vi "Process.vi"(8 "error in (no error)":errorcluster, 10 "pound in":refnum<class "Pound.lvclass">, 11 "Qbus in":refnum<class "Qbus.lvclass">) -> (0 "error out":errorcluster)   [LabVIEW 2017, in "DataAccumulator.lvlib"]
doc: "This process combines waveforms from successive acquisitions to achieve the data block sizes configured in Systems Manager. The combined waveforms make up the data sets on which the Analysis process calculates features and spectral bands. Later, the Trigger and Alarm processes evaluate those feature values for operating state and alarm transitions."
uses:
  <vilib>/addons/InsightCM/Devices/Shared/Common/DataAccumulator/DataAccumulator.lvlib
  <vilib>/addons/Qbus/Qbus.lvclass
  <vilib>/NI/Software Watchdog/Pound/Pound.lvclass
  <vilib>/addons/TimerProcess/controls/taskType.ctl
  <vilib>/addons/InsightCM/Devices/Shared/Common/DataFlow/controls/Type.ctl
  <vilib>/addons/InsightCM/Devices/Shared/Common/DataAccumulator/controls/DataStoreOps.ctl
  <vilib>/addons/TraceLogger/TraceLogger.lvlib
  <vilib>/NI/Software Watchdog/Watchdog/Watchdog.lvclass
  <vilib>/addons/InsightCM/Devices/Shared/Common/DVRBuffer/DVRBuffer.lvlib
  <vilib>/addons/InsightCM/Devices/Shared/Common/DataFlow/DataFlow.lvlib
  <vilib>/addons/InsightCM/Utilities/GlobalConfiguration/GlobalConfiguration.lvlib
  <vilib>/addons/TimerProcess/TimerProcess.lvlib
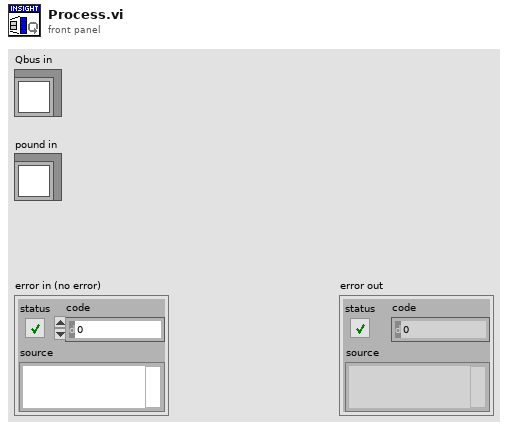
[diagram p1: front panel]
types:
  T1 = typedef "TimerProcess.lvlib/taskType.ctl" = enum16{"single", "repeat"}
  T2 = typedef "DataFlow.lvlib/Type.ctl" = enum16{"High Rate", "Low Rate", "Burst Mode"}
  T3 = typedef "DataAccumulator.lvlib/DataStoreOps.ctl" = enum16{"Reset", "Init", "Clear", "SetWfms", "GetWfms"}
  T4 = typedef "DataFlow.lvlib/Data.ctl" = cluster{"DataGroup":string, "Waveforms":T5, "Map":T6, "Type":T2}
  T5 = typedef "wfmSGL_DVR.ctl" = refnum<data-value>
  T6 = typedef "PointValueMap.lvlib/PointMap.ctl" = refnum<data-value>
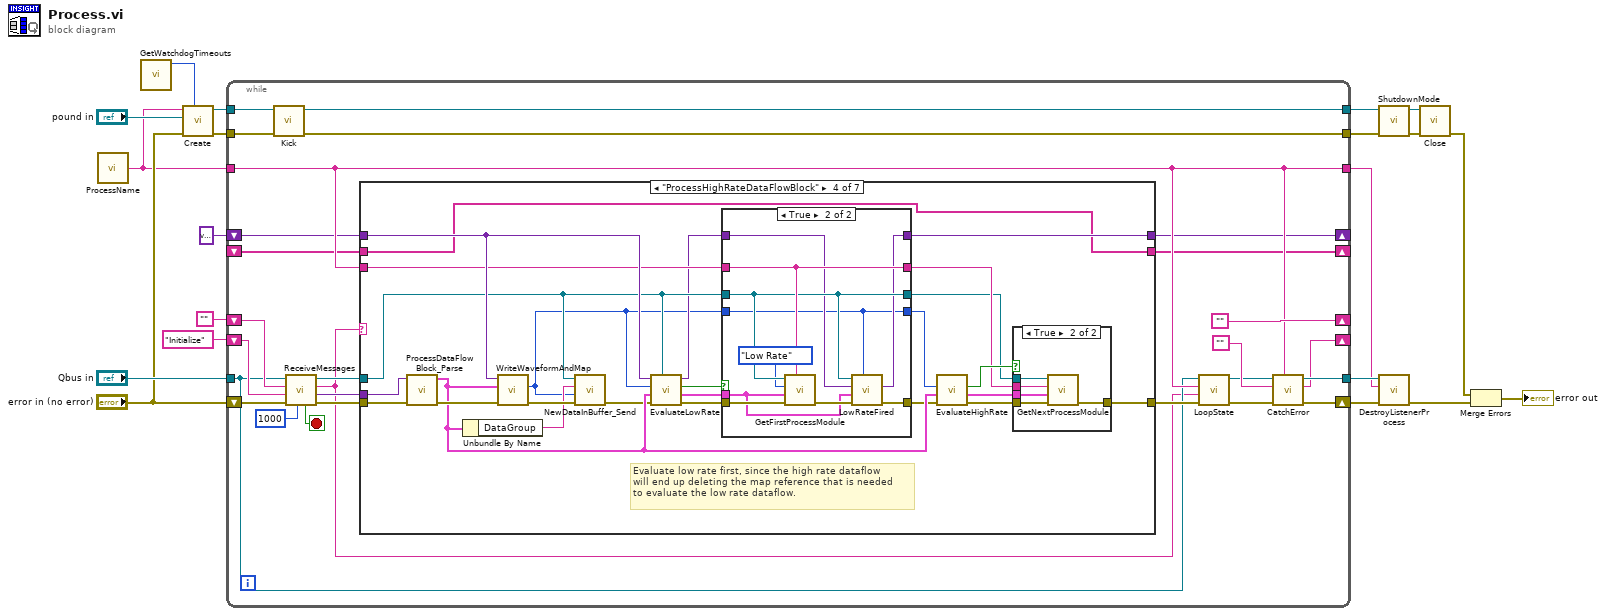
[diagram p0: block diagram]
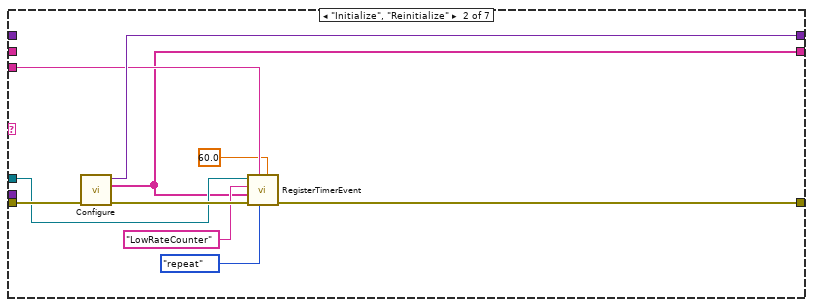
[diagram p3: hidden frame]
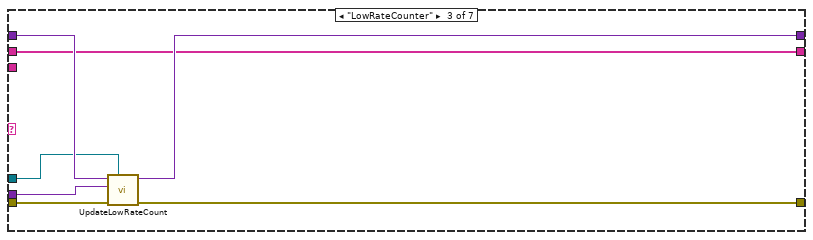
[diagram p4: hidden frame]
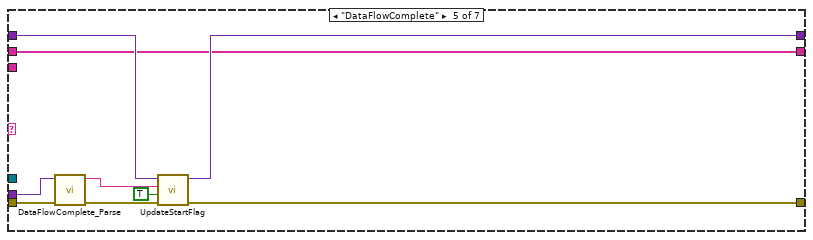
[diagram p7: hidden frame]
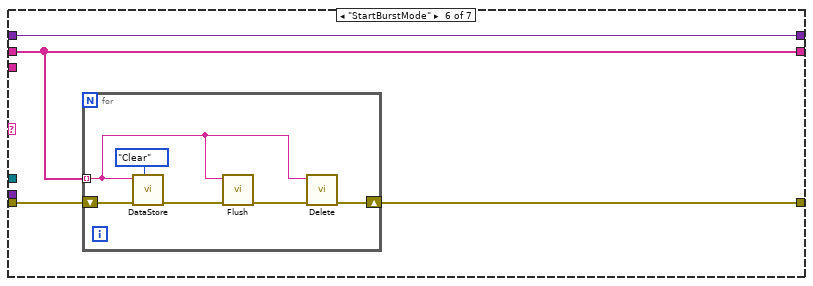
[diagram p8: hidden frame]
diagram:
  n1 = call <vilib>:"ProcessName.vi"() -> ("process name"=w1:string)  [unwired: 5 in]
  n2 = call <vilib>:"GetWatchdogTimeouts.vi"() -> ("software timeout"=w2:u32)  [unwired: 10 in, 1 out]
  n3 = call <vilib>:"Create.vi"("Execution Timeout (ms)"=w2, "error in (no error)"="error in (no error)", "Pound"="pound in", "Name"=w1) -> ("error out"=w10:errorcluster, "Watchdog"=w15:refnum<data-value>)  [unwired: 6 in]
  n4 = while {
    shift-right: [""] -> _
    shift-left: "" -> [w46]
    tunnel: "Qbus in" -> [w34]
    tunnel: w1 -> [w35]
    tunnel: [w39] -> w18
    tunnel: [w35] -> w17
    shift-right: [w37] -> _
    shift-left: "Initialize" -> [w41]
    tunnel: w15 -> [w33]
    tunnel: [w32] -> w12
    tunnel: w10 -> [w31]
    tunnel: [w29] -> w9
    shift-right: [w26] -> _
    shift-left: variant -> [w25]
    shift-right: [w40] -> w19
    shift-left: "error in (no error)" -> [w30]
    shift-right: [w22] -> _
    shift-left: _ -> [w21]
    stop <- w47 stop-if-true
    n5 = call <vilib>:"Kick.vi"("error in (no error)"=w31, "Watchdog"=w33) -> ("error out"=w29:errorcluster, "Watchdog"=w32:refnum<data-value>)  [unwired: 8 in]
    n6 = call <vilib>:"ReceiveMessages.vi"("timeout (1000)"=1000 ("milliseconds to wait"), "error in (no error)"=w30, "priority action"=w41, "default action"=w46, "Qbus in"=w34) -> ("error out"=w45:errorcluster, "message value"=w42:variant, "action"=w28:string, "Qbus out"=w43:refnum<class "Qbus.lvclass">, "exit"=w47:bool)  [unwired: 2 in]
    n7 = case shown="\"ProcessHighRateDataFlowBlock\"" w28 {
      tunnel: w45 -> [w50 w60 w63 w91 w118 w125 w135]
      tunnel: w43 -> [_ w56 w62 w75 _ _ _]
      tunnel: [w50 w57 w65 w76 w121 w124 w135] -> w36
      tunnel: w42 -> [_ _ w64 w90 w116 _ _]
      tunnel: w35 -> [_ w55 _ w81 _ _ _]
      tunnel: [w49 w59 w66 w74 w120 w126 w134] -> w26
      tunnel: w25 -> [w49 _ w67 w87 w122 w126 w134]
      tunnel: [w48 w51 w61 w68 w114 w123 w133] -> w22
      tunnel: w21 -> [w48 _ w61 w68 w114 w123 w133]
      frame "", Default {
      }
      frame "Initialize", "Reinitialize" {
        n8 = call <vilib>:"Configure.vi"("error in (no error)"=w60) -> ("error out"=w58:errorcluster, "groups"=w51:string[], "config"=w59:variant)  [unwired: 8 in]
        n9 = call <vilib>:"RegisterTimerEvent.vi"("interval (sec)"=60.0, "type"=taskType."repeat", "process name"=w55, "error in (no error)"=w58, "callback value"=w51, "callback action"="LowRateCounter", "qbus in"=w56) -> ("error out"=w57:errorcluster)  [unwired: 3 in, 1 out]
      }
      frame "LowRateCounter" {
        n10 = call <vilib>:"UpdateLowRateCount.vi"("Qbus in"=w62, "error in (no error)"=w63, "message value"=w64, "config"=w67) -> ("error out"=w65:errorcluster, "config out"=w66:variant)  [unwired: 6 in]
      }
      frame "ProcessHighRateDataFlowBlock" {
        # "Evaluate low rate first, since the high rate dataflow\nwill end up deleting the map reference that is needed\nto evaluate the low rate dataflow."
        n11 = call <vilib>:"ProcessDataFlowBlock_Parse.vi"("error in (no error)"=w91, "body"=w90) -> ("error out"=w88:errorcluster, "data"=w80:T4)  [unwired: 8 in]
        n12 = Unbundle By Name(w80) -> ("DataGroup"=w89:string)
        n13 = call <vilib>:"WriteWaveformAndMap.vi"("error in (no error)"=w88, "data"=w80, "config"=w87) -> ("error out"=w92:errorcluster, "block number"=w70:u32)  [unwired: 6 in, 1 out]
        n14 = call <vilib>:"NewDataInBuffer_Send.vi"("error in (no error)"=w92, "buffer location"=w70, "data group"=w89, "Qbus in"=w75) -> ("error out"=w79:errorcluster)  [unwired: 6 in, 1 out]
        n15 = call <vilib>:"EvaluateLowRate.vi"("Qbus"=w75, "error in (no error)"=w79, "data"=w80, "new block number"=w70, "config"=w87) -> ("error out"=w84:errorcluster, "new data"=w85:T4, "fire low rate data flow"=w86:bool, "config out"=w73:variant)  [unwired: 3 in]
        n16 = case shown="True" w86 {
          tunnel: w85 -> [_ w110]
          tunnel: w84 -> [w103 w113]
          tunnel: [w103 w111] -> w78
          tunnel: w75 -> [w100 w108]
          tunnel: w81 -> [w101 w109]
          tunnel: [w102 w106] -> w74
          tunnel: w73 -> [w102 w107]
          tunnel: [w101 w109] -> w72
          tunnel: [w100 w108] -> w71
          tunnel: w70 -> [w99 w105]
          tunnel: [w99 w105] -> w69
          frame False {
          }
          frame True {
            n17 = call <vilib>:"GetFirstProcessModule.vi"("originator"=w109, "error in (no error)"=w113, "data"=w110, "type"=Type."Low Rate", "Qbus in"=w108) -> ("error out"=w112:errorcluster)  [unwired: 5 in, 1 out]
            n18 = call <vilib>:"LowRateFired.vi"("new block number"=w105, "error in (no error)"=w112, "new data"=w110, "config in"=w107, "Qbus"=w108) -> ("error out"=w111:errorcluster, "config out"=w106:variant)  [unwired: 5 in]
          }
        }
        n19 = call <vilib>:"EvaluateHighRate.vi"("error in (no error)"=w78, "data in"=w80, "block number"=w69) -> ("error out"=w77:errorcluster, "data out"=w83:T4, "complete"=w82:bool)  [unwired: 6 in]
        n20 = case shown="True" w82 {
          tunnel: w72 -> [_ w98]
          tunnel: [w93 w95] -> w76
          tunnel: w71 -> [_ w97]
          tunnel: w77 -> [w93 w94]
          tunnel: w83 -> [_ w96]
          frame False {
          }
          frame True {
            n21 = call <vilib>:"GetNextProcessModule.vi"("error in (no error)"=w94, "data"=w96, "source"=w98, "Qbus in"=w97) -> ("error out"=w95:errorcluster)  [unwired: 6 in, 1 out]
          }
        }
      }
      frame "DataFlowComplete" {
        n22 = call <vilib>:"DataFlowComplete_Parse.vi"("error in (no error)"=w118, "body"=w116) -> ("error out"=w117:errorcluster, "group"=w119:string)  [unwired: 8 in]
        n23 = call <vilib>:"UpdateStartFlag.vi"("error in (no error)"=w117, "BlkComplete"=TRUE, "group"=w119, "config"=w122) -> ("error out"=w121:errorcluster, "config"=w120:variant)  [unwired: 6 in]
      }
      frame "StartBurstMode" {
        n24 = for {
          shift-right: [w128] -> w124
          shift-left: w125 -> [w131]
          tunnel: w123 -> [w127] mode=indexing
          n25 = call <vilib>:"DataStore.vi"("operation"=DataStoreOps."Clear", "error in (no error)"=w131, "group"=w127) -> ("error out"=w130:errorcluster)  [unwired: 7 in, 1 out]
          n26 = call <vilib>:"Flush.vi"("error in (no error)"=w130, "name"=w127) -> ("error out"=w129:errorcluster)  [unwired: 9 in]
          n27 = call <vilib>:"Delete.vi"("error in (no error)"=w129, "name"=w127) -> ("error out"=w128:errorcluster)  [unwired: 9 in]
        }
      }
      frame "Exit" {
      }
    }
    n28 = call <vilib>:"LoopState.vi"("error in (no error)"=w36, "loop action"=w28, "process name"=w35, "Qbus in"=w34) -> ("error out"=w24:errorcluster, "Qbus out"=w23:refnum<class "Qbus.lvclass">)  [unwired: 6 in]
    n29 = call <vilib>:"CatchError.vi"("source"=w35, "error in (no error)"=w24, "next action in"="", "Qbus in"=w23) -> ("error out"=w40:errorcluster, "next action out"=w37:string, "Qbus out"=w39:refnum<class "Qbus.lvclass">)  [unwired: 5 in]
  }
  n30 = call <vilib>:"ShutdownMode.vi"("error in (no error)"=w9, "Watchdog"=w12) -> ("error out"=w11:errorcluster, "Watchdog"=w13:refnum<data-value>)  [unwired: 8 in]
  n31 = call <vilib>:"DestroyListenerProcess.vi"("error in (no error)"=w19, "process name"=w17, "Qbus in"=w18) -> ("error in (no error)"=w8:errorcluster)  [unwired: 7 in, 1 out]
  n32 = call <vilib>:"Close.vi"("error in (no error)"=w11, "Watchdog"=w13) -> ("error out"=w7:errorcluster)  [unwired: 9 in]
  n33 = Merge Errors(w7, w8) -> (→"error out":errorcluster)
